vi "log_duilie.vi"(5 "LabVIEW Web Service Request":refnum<class "Web Request.lvclass"> caption="LabVIEW Web服务请求", 7 "type":string, 8 "action":string, 9 "user":string, 11 "yw":string) -> ()   [LabVIEW 2017, in "Lib_code.lvlib"]
uses:
  Lib_code.lvlib
  <vilib>/wsapi/Web Request.lvclass
panel:
  in  "variable name":string(combo)="REMOTE_ADDR" caption="变量名称"
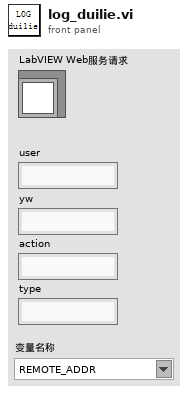
[diagram p1: front panel]
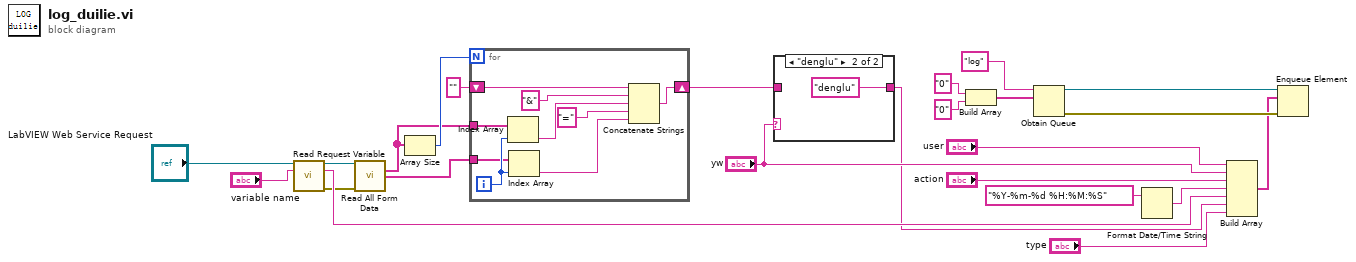
[diagram p0: block diagram]
diagram:
  n1 = call <vilib>:"Read Request Variable.vi"("LabVIEW Web Service Request"="LabVIEW Web Service Request", "variable name"="variable name") -> ("LabVIEW Web Service Request out"=w6:refnum<class "Web Request.lvclass">, "value"=w11:string, "error out"=w5:errorcluster)  [unwired: 11 in]
  n2 = call <vilib>:"Read All Form Data.vi"("LabVIEW Web Service Request"=w6, "error in (no error)"=w5) -> ("Key"=w8:string[], "Value"=w7:string[])  [unwired: 9 in, 3 out]
  n3 = Array Size(array=w8) -> (size(s)=w9:i32)
  n4 = for {
    N: w9 -> [_]
    tunnel: w8 -> [w32]
    tunnel: w7 -> [w31]
    shift-right: [w29] -> w1
    shift-left: "" -> [w30]
    i -> [w33]
    n5 = Index Array(array=w32, index=w33) -> (element=w27:string)
    n6 = Index Array(array=w31, index=w33) -> (element=w25:string)
    n7 = Concatenate Strings(w30, "&" ("字符串"), w27, "=" ("字符串"), w25) -> (w29:string)
  }
  n8 = case shown="\"denglu\"" "yw" {
    tunnel: [w34 "denglu"] -> w2
    tunnel: w1 -> [w34 _]
    frame "假", Default {
    }
    frame "denglu" {
    }
  }
  n9 = Build Array("0" ("元素"), "0" ("元素")) -> (w21:string[])
  n10 = Obtain Queue(name (unnamed)="log" ("名称（未命名）"), element data type=w21) -> (queue out=w20:refnum<queue>, error out=w19:errorcluster)  [unwired: 3 in, 1 out]
  n11 = Format Date/Time String(time format string (%c)="%Y-%m-%d %H:%M:%S" ("时间格式字符串(%c)")) -> (date/time string=w14:string)  [unwired: 2 in]
  n12 = Build Array("user", "yw", "action", w14, w11, w2, "type") -> (w16:string[])
  n13 = Enqueue Element(queue=w20, element=w16, error in (no error)=w19) -> ()  [unwired: 1 in, 3 out]
